vi "FPGAcode4_multipleArrays.vi"() -> ()   [LabVIEW 2015]
uses:
  Limits_In.ctl
  Detector_Cluster.ctl
  <vilib>/Platform/TimedLoop/XDataNode/timing_clust.ctl
  <vilib>/Platform/TimedLoop/XDataNode/nitl_modes.ctl
  <vilib>/Platform/TimedLoop/XDataNode/wakeup.ctl
  Correlations.ctl
  <vilib>/rvi/Emulation/niFpgaSctlEmulationGetInTimedLoop.vi
  <vilib>/rvi/Emulation/niFpgaEmulationReportErrorSimple.vi
  <vilib>/rvi/Emulation/niFpgaGetClockAttributes.vi
  <vilib>/rvi/Emulation/niFpgaCriticalErrorInLSC.vi
  <vilib>/rvi/eio/common/nirviEmuTemplateMethod_errors.vi
  <vilib>/rvi/Emulation/niFpgaEmulationIsFPGAContextNoSignature.vi
  <vilib>/rvi/DataTransferAndStorage/Container/Common/niFpgaContainerGetUniqueNameForEmu.vi
  <vilib>/rvi/eio/common/nirviEmuReportErrorAndStop.vi
  <vilib>/rvi/Emulation/niFpgaProcessEmulError.vi
  <vilib>/Platform/TimedLoop/XDataNode/XDataNode.xnode
  <vilib>/eio/EIONode/EIONode.xnode
  <vilib>/rvi/DataTransferAndStorage/Container/XNode/niFpgaContainer.xnode
  <vilib>/rvi/DataTransferAndStorage/Handshake/Emulation/niFpgaHandshakeEmulation.vi
  <vilib>/Platform/TimedLoop/XDataNode/XDNodeRunTimeDep.lvlib
panel:
  in  "Charge Error Factor":fxp<+,32,0>=0.19999999995343387 format="%_2g"
  in  "Calibrate":bool=TRUE
  in  "Limits":T1={"High Charge Limit"=4.54747350780585e-13, "Low Charge Limit"=0.0, "High Velocity Limit"=262143.0, "Low Velocity Limit"=0.0, "High Mass Limit"=7.27595761248936e-12, "Low Mass Limit"=0.0, "High Voltage"=2200000.0}
  in  "One Shot":bool
  in  "Threshold Factor":fxp<+/-,32,16>=1.149993896484375 format="%.2g"
  in  "Armed":bool
  in  "User Trigger Distance":fxp<+/-,34,18> format="%.3g"
  in  "User Trigger?":bool
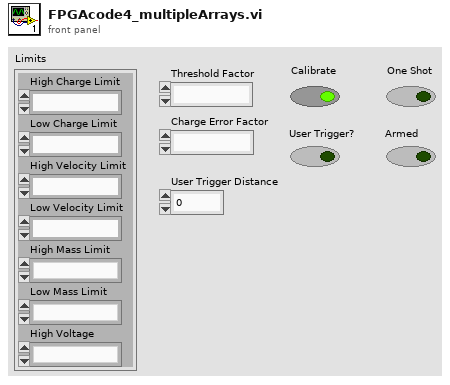
[diagram p1: front panel]
types:
  T1 = typedef "Limits_In.ctl" = cluster{"High Charge Limit":fxp<+,32,-41>, "Low Charge Limit":fxp<+,32,-41>, "High Velocity Limit":fxp<+,18,18>, "Low Velocity Limit":fxp<+,18,18>, "High Mass Limit":fxp<+,32,-37>, "Low Mass Limit":fxp<+,32,-37>, "High Voltage":fxp<+,32,22>}
  T2 = cluster{"[0]":fxp<+,16,1>, "[1]":fxp<+,16,1>, "[2]":fxp<+,16,1>, "[3]":fxp<+,16,1>, "[4]":fxp<+,16,1>, "[5]":fxp<+,16,1>, "[6]":fxp<+,16,1>, "[7]":fxp<+,16,1>, "[8]":fxp<+,16,1>, "[9]":fxp<+,16,1>, "[10]":fxp<+,16,1>}
  T3 = cluster{"[0]":i32, "[1]":i32, "[2]":i32, "[3]":i32, "[4]":i32, "[5]":i32, "[6]":i32, "[7]":i32, "[8]":i32, "[9]":i32, "[10]":i32}
  T4 = cluster{"[0]":cluster{"Detector Max Speed Count":i32, "Detector Min Speed Count":i32, "Gap Max Speed Count":i32, "Gap Min Speed Count":i32}, "[1]":cluster{"Detector Max Speed Count":i32, "Detector Min Speed Count":i32, "Gap Max Speed Count":i32, "Gap Min Speed Count":i32}, "[2]":cluster{"Detector Max Speed Count":i32, "Detector Min Speed Count":i32, "Gap Max Speed Count":i32, "Gap Min Speed Count":i32}, "[3]":cluster{"Detector Max Speed Count":i32, "Detector Min Speed Count":i32, "Gap Max Speed Count":i32, "Gap Min Speed Count":i32}, "[4]":cluster{"Detector Max Speed Count":i32, "Detector Min Speed Count":i32, "Gap Max Speed Count":i32, "Gap Min Speed Count":i32}, "[5]":cluster{"Detector Max Speed Count":i32, "Detector Min Speed Count":i32, "Gap Max Speed Count":i32, "Gap Min Speed Count":i32}, "[6]":cluster{"Detector Max Speed Count":i32, "Detector Min Speed Count":i32, "Gap Max Speed Count":i32, "Gap Min Speed Count":i32}, "[7]":cluster{"Detector Max Speed Count":i32, "Detector Min Speed Count":i32, "Gap Max Speed Count":i32, "Gap Min Speed Count":i32}, "[8]":cluster{"Detector Max Speed Count":i32, "Detector Min Speed Count":i32, "Gap Max Speed Count":i32, "Gap Min Speed Count":i32}, "[9]":cluster{"Detector Max Speed Count":i32, "Detector Min Speed Count":i32, "Gap Max Speed Count":i32, "Gap Min Speed Count":i32}, "[10]":cluster{"Detector Max Speed Count":i32, "Detector Min Speed Count":i32, "Gap Max Speed Count":i32, "Gap Min Speed Count":i32}}
  T5 = cluster{cluster{"[0]":i32, "[1]":i32, "[2]":i32, "[3]":i32, "[4]":i32, "[5]":i32, "[6]":i32, "[7]":i32, "[8]":i32, "[9]":i32, "[10]":i32}, cluster{"[0]":i32, "[1]":i32, "[2]":i32, "[3]":i32, "[4]":i32, "[5]":i32, "[6]":i32, "[7]":i32, "[8]":i32, "[9]":i32, "[10]":i32}, cluster{"[0]":i32, "[1]":i32, "[2]":i32, "[3]":i32, "[4]":i32, "[5]":i32, "[6]":i32, "[7]":i32, "[8]":i32, "[9]":i32, "[10]":i32}, cluster{"[0]":i32, "[1]":i32, "[2]":i32, "[3]":i32, "[4]":i32, "[5]":i32, "[6]":i32, "[7]":i32, "[8]":i32, "[9]":i32, "[10]":i32}}
  T6 = cluster{"Distance to PSU":fxp<+/-,64,37>, "Distance to end of PSU":fxp<+/-,64,37>, "Distance to DCS 2":fxp<+/-,64,37>, "Distance to DCS 1":fxp<+/-,64,37>, "Distance to front of LEIL Chamber":fxp<+/-,64,37>}
  T7 = typedef "Detector_Cluster.ctl" = cluster{"Det 1":i32, "Det 2":i32}
  T8 = cluster{"Filter 1":T7, "Filter 2":T7, "Filter 3":T7, "Filter 4":T7}
  T9 = cluster{"Detector Max Speed Count":i32, "Detector Min Speed Count":i32, "Gap Max Speed Count":i32, "Gap Min Speed Count":i32}[]
  T10 = cluster{"Filter 1":T7, "Filter 2":T7, "Filter 3":T7, "Filter 4":T7}[]
  T11 = typedef "XDNodeRunTimeDep.lvlib/timing_clust.ctl" = cluster{"Expected End [f-1]":u64, "Actual End [f-1]":u64, "Finished Late? [f-1]":bool, "Expected End [i-1]":u64, "Actual End [i-1]":u64, "Finished Late? [i-1]":bool, "Expected Start [i]":u64, "Actual Start [i]":u64, "Expected Start [f]":u64, "Actual Start [f]":u64, "Source Name":string, "Structure Name":string, "Period":i64, "Deadline":i64, "Offset":i64, "Start":i64, "Priority":i32, "Timeout":i32, "Mode":T12, "Wakeup Reason":T13, "Error":errorcluster, "Source Type":string, "Secondary Source Type":string, "Global End Time":u64, "Global Start Time":u64, "Frame Duration":u64, "Iteration Duration":u64, "Assigned CPU":i32, "I/O Scan Engine Mode":u32}
  T12 = typedef "XDNodeRunTimeDep.lvlib/nitl_modes.ctl" = enum32{"No Change", "Process missed periods, maintain original phase", "Discard missed periods, maintain original phase", "Process missed periods, ignore original phase", "Discard missed periods, ignore original phase"}
  T13 = typedef "XDNodeRunTimeDep.lvlib/wakeup.ctl" = enum32{"Normal", "Aborted", "Asynchronous wakeup", "Timing source error", "Timed loop error", "Timeout"}
  T14 = cluster{"IO Module\\AI 0":i16, "IO Module\\AI 1":i16}
  T15 = cluster{"First Detector Count":i32, "Detector Gap Count":i32, "Second Detector Count":i32, "Second Detector Final Count":i32}
  T16 = typedef "Correlations.ctl" = cluster{"First Correlation":i32, "Latest Correlation":i32}
  T17 = cluster{"Data":fxp<+/-,40,32>, "Data":fxp<+/-,40,32>}
  T18 = cluster{cluster{"Data":i16, "Data":i16}, cluster{"Det 1":i16, "Det 2":i16}, cluster{"Det 1":i16, "Det 2":i16}, cluster{"Det 1":i16, "Det 2":i16}}
  T19 = cluster{cluster{"Det 1":i16, "Det 2":i16}, cluster{"Det 1":i16, "Det 2":i16}, cluster{"Det 1":i16, "Det 2":i16}, cluster{"Det 1":i16, "Det 2":i16}}
  T20 = cluster{"Distance to PSU":fxp<+/-,64,69>, "Distance to end of PSU":fxp<+/-,64,69>, "Distance to DCS 2":fxp<+/-,64,69>, "Distance to DCS 1":fxp<+/-,64,69>, "Distance to front of LEIL Chamber":fxp<+/-,64,69>}
  T21 = cluster{"Distance to PSU":i32, "Distance to end of PSU":i32, "Distance to DCS 2":i32, "Distance to DCS 1":i32, "Distance to front of LEIL Chamber":i32}
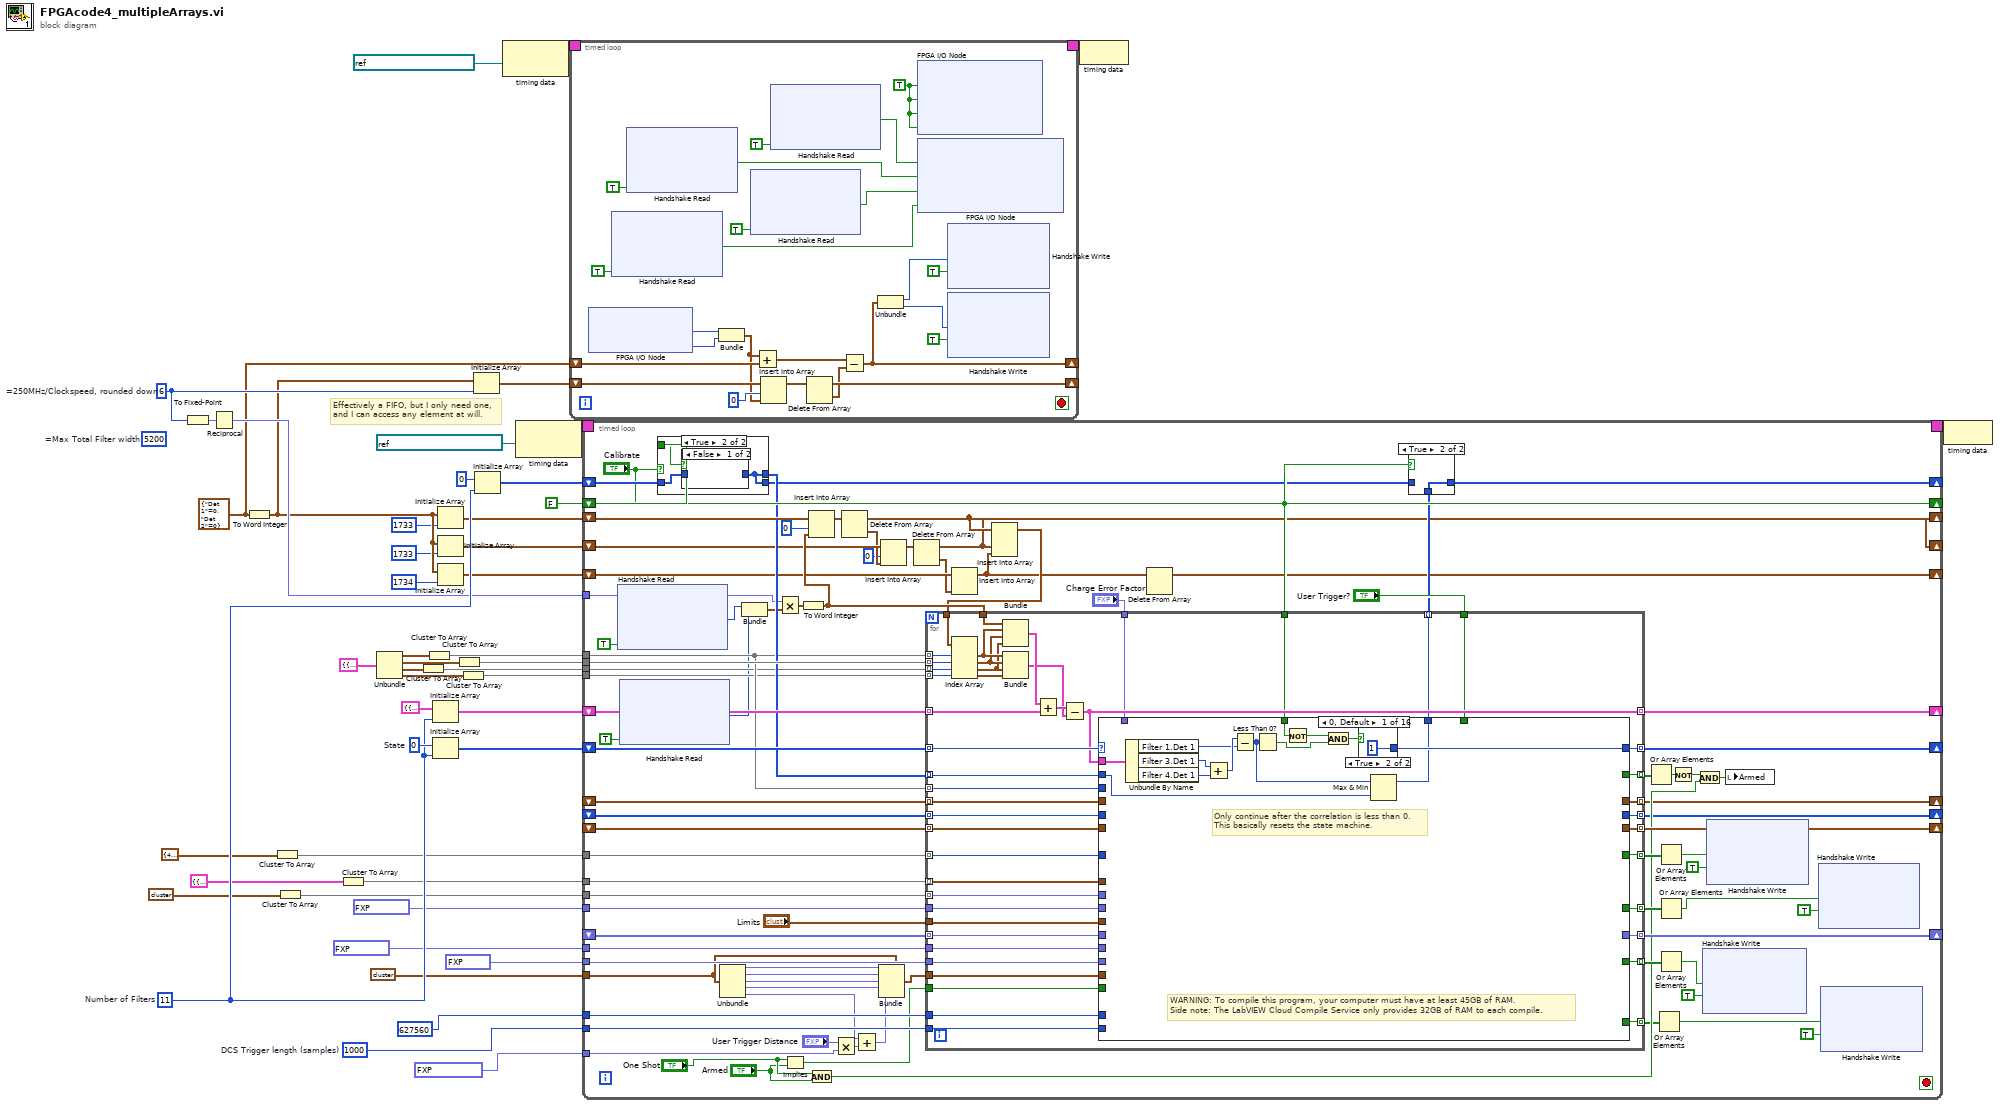
[diagram p0: block diagram]
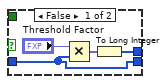
[diagram p2: hidden frame]
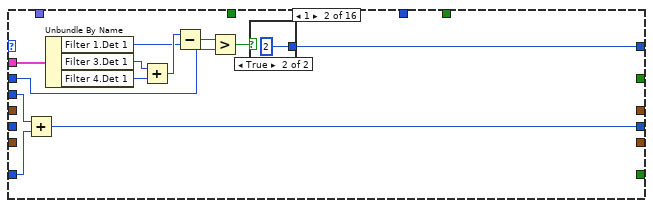
[diagram p6: hidden frame]
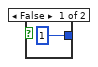
[diagram p7: hidden frame]
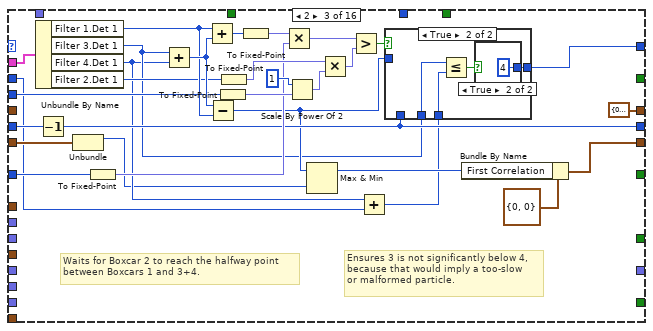
[diagram p8: hidden frame]
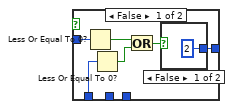
[diagram p9: hidden frame]
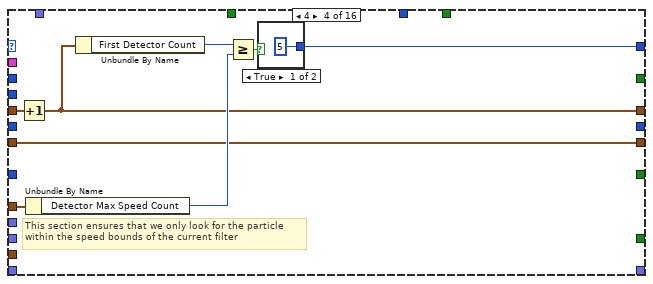
[diagram p12: hidden frame]
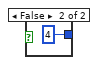
[diagram p13: hidden frame]
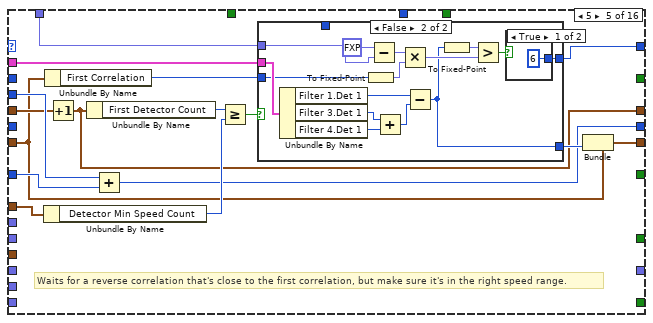
[diagram p14: hidden frame]
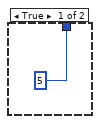
[diagram p15: hidden frame]
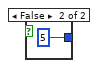
[diagram p16: hidden frame]
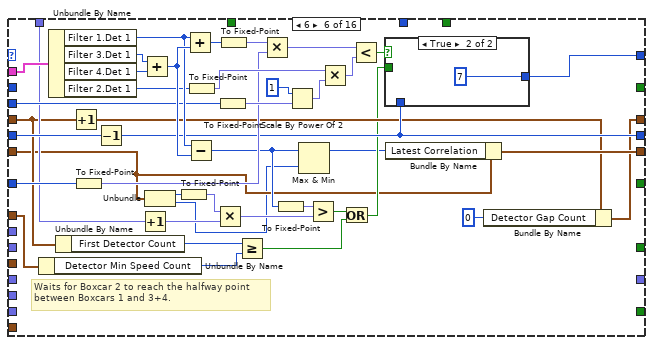
[diagram p17: hidden frame]
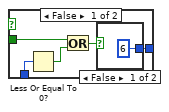
[diagram p18: hidden frame]
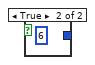
[diagram p19: hidden frame]
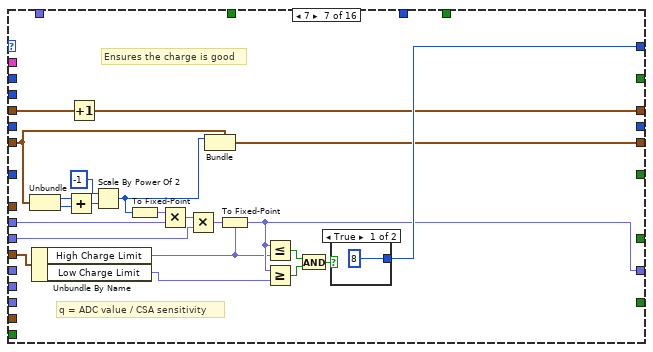
[diagram p20: hidden frame]
diagram:
  w40 = u8 6  # =250MHz/Clockspeed, rounded down
  (unwired) 5200  # =Max Total Filter width
  w10 = u16 1000  # DCS Trigger length (samples)
  w7 = T7 {"Det 1"=0, "Det 2"=0} ("Detectors")
  w48 = u8 0  # State
  w45 = 11  # Number of Filters
  # "Effectively a FIFO, but I only need one,\nand I can access any element at will."
  n1 = To Fixed-Point(number=w40) -> (fixed-point=w42:fxp<+,8,8>)  [unwired: 1 in]
  n2 = Reciprocal(x=w42) -> (1/x=w25:fxp<+,9,1>)
  n3 = To Word Integer(number=w7) -> (16bit integer=w6:cluster{"Det 1":i16, "Det 2":i16})
  n4 = Cluster To Array(cluster=T3 {"[0]"=4000, "[1]"=2359, "[2]"=1391, "[3]"=820, "[4]"=484, "[5]"=285, "[6]"=168, "[7]"=99, "[8]"=59, "[9]"=35, "[10]"=20}) -> (array=w18:i32[])
  n5 = Cluster To Array(cluster=T2 {"[0]"=0.000823974609375, "[1]"=0.000823974609375, "[2]"=0.000823974609375, "[3]"=0.000823974609375, "[4]"=0.000823974609375, "[5]"=0.00152587890625, "[6]"=0.003265380859375, "[7]"=0.007080078125, "[8]"=0.015869140625, "[9]"=0.03704833984375, "[10]"=0.100006103515625} ("cluster 3")) -> (array=w16:fxp<+,16,1>[])
  n6 = Cluster To Array(cluster=T4 {"[0]"={"Detector Max Speed Count"=42000, "Detector Min Speed Count"=84000, "Gap Max Speed Count"=78000, "Gap Min Speed Count"=156000}, "[1]"={"Detector Max Speed Count"=21477, "Detector Min Speed Count"=42953, "Gap Max Speed Count"=39885, "Gap Min Speed Count"=79770}, "[2]"={"Detector Max Speed Count"=10982, "Detector Min Speed Count"=21964, "Gap Max Speed Count"=20395, "Gap Min Speed Count"=40790}, "[3]"={"Detector Max Speed Count"=5616, "Detector Min Speed Count"=11231, "Gap Max Speed Count"=10429, "Gap Min Speed Count"=20858}, "[4]"={"Detector Max Speed Count"=2872, "Detector Min Speed Count"=5743, "Gap Max Speed Count"=5333, "Gap Min Speed Count"=10666}, "[5]"={"Detector Max Speed Count"=1468, "Detector Min Speed Count"=2937, "Gap Max Speed Count"=2727, "Gap Min Speed Count"=5454}, "[6]"={"Detector Max Speed Count"=751, "Detector Min Speed Count"=1502, "Gap Max Speed Count"=1394, "Gap Min Speed Count"=2789}, "[7]"={"Detector Max Speed Count"=384, "Detector Min Speed Count"=768, "Gap Max Speed Count"=713, "Gap Min Speed Count"=1426}, "[8]"={"Detector Max Speed Count"=196, "Detector Min Speed Count"=393, "Gap Max Speed Count"=365, "Gap Min Speed Count"=729}, "[9]"={"Detector Max Speed Count"=100, "Detector Min Speed Count"=201, "Gap Max Speed Count"=186, "Gap Min Speed Count"=373}, "[10]"={"Detector Max Speed Count"=51, "Detector Min Speed Count"=103, "Gap Max Speed Count"=95, "Gap Min Speed Count"=191}} ("cluster 2")) -> (array=w17:T9)
  n7 = Unbundle(T5 {{"[0]"=1200, "[1]"=1200, "[2]"=1200, "[3]"=1200, "[4]"=1200, "[5]"=650, "[6]"=306, "[7]"=140, "[8]"=62, "[9]"=26, "[10]"=10}, {"[0]"=5200, "[1]"=3559, "[2]"=2591, "[3]"=2020, "[4]"=1684, "[5]"=935, "[6]"=474, "[7]"=240, "[8]"=122, "[9]"=62, "[10]"=30}, {"[0]"=5800, "[1]"=4159, "[2]"=3191, "[3]"=2620, "[4]"=2284, "[5]"=1260, "[6]"=627, "[7]"=310, "[8]"=153, "[9]"=75, "[10]"=35}, {"[0]"=6400, "[1]"=4759, "[2]"=3791, "[3]"=3220, "[4]"=2884, "[5]"=1585, "[6]"=780, "[7]"=380, "[8]"=184, "[9]"=88, "[10]"=40}} ("output cluster")) -> (w38:T3, w37:T3, w36:T3, w35:T3)
  n8 = Cluster To Array(cluster=w36) -> (array=w22:i32[])
  n9 = Cluster To Array(cluster=w38) -> (array=w24:i32[])
  n10 = Initialize Array(T8 {"Filter 1"={"Det 1"=0, "Det 2"=0}, "Filter 2"={"Det 1"=0, "Det 2"=0}, "Filter 3"={"Det 1"=0, "Det 2"=0}, "Filter 4"={"Det 1"=0, "Det 2"=0}} ("cluster"), w45) -> (w20:T10)
  n11 = Initialize Array(w48, w45) -> (w19:u8[])
  n12 = Initialize Array(w6, 1733 ("dimension size")) -> (w26:cluster{"Det 1":i16, "Det 2":i16}[])
  n13 = Initialize Array(w6, 1733 ("dimension size")) -> (w5:cluster{"Det 1":i16, "Det 2":i16}[])
  n14 = Initialize Array(w6, 1734 ("dimension size")) -> (w4:cluster{"Det 1":i16, "Det 2":i16}[])
  n15 = Cluster To Array(cluster=w37) -> (array=w23:i32[])
  n16 = Cluster To Array(cluster=w35) -> (array=w21:i32[])
  n17 = Initialize Array(w6, w40) -> (w41:cluster{"Det 1":i16, "Det 2":i16}[])
  n18 = Initialize Array(0 ("Thresholds in"), w45) -> (w27:i32[])
  n19 = node-c288(refnum<k21> "IO Module\\Data Clock" ("Source Name")) -> (w44:T11)
  n20 = node-c288(refnum<k21> "40 MHz Onboard Clock" ("Source Name")) -> (w30:T11)
  n21 = timed-loop {
    timing: w44 -> [_]
    timing-out: [_] -> w43
    shift-right: [w62] -> _
    shift-left: w7 -> [w71]
    shift-right: [w64] -> _
    shift-left: w41 -> [w69]
    stop <- _ stop-if-true
    w49 = TRUE ("IO Module\\PFI Enable")
    n22 = xnode "FPGA I/O Node"() -> ("IO Module\\AI 0"=w68:i16, "IO Module\\AI 1"=w67:i16)  [unwired: 2 in, 2 out]
    n23 = xnode ("Handshake Read")("Ready for Output"=TRUE) -> ("Data"=w57:bool)  [unwired: 1 in, 2 out]
    n24 = xnode ("Handshake Read")("Ready for Output"=TRUE) -> ("Data"=w53:bool)  [unwired: 1 in, 2 out]
    n25 = Bundle("IO Module\\AI 0"=w68, "IO Module\\AI 1"=w67) -> (w66:T14)  [unwired: 1 in]
    n26 = xnode ("Handshake Read")("Ready for Output"=TRUE) -> ("Data"=w56:bool)  [unwired: 1 in, 2 out]
    n27 = Add(x=w66, y=w71) -> (x+y=w70:T7)
    n28 = Insert Into Array(array=w69, index=0, new element=w66) -> (w65:cluster{"Det 1":i16, "Det 2":i16}[])
    n29 = xnode ("Handshake Read")("Ready for Output"=TRUE) -> ("Data"=w50:bool)  [unwired: 1 in, 2 out]
    n30 = Delete From Array(array=w65) -> (deleted portion=w63:cluster{"Det 1":i16, "Det 2":i16}, array with subset deleted=w64:cluster{"Det 1":i16, "Det 2":i16}[])  [unwired: 2 in]
    n31 = Subtract(x=w70, y=w63) -> (x-y=w62:T7)
    n32 = Unbundle(w62) -> ("Det 1"=w60:i32, "Det 2"=w58:i32)
    n33 = xnode "FPGA I/O Node"("IO Module\\PFI 0 WE"=w49, "IO Module\\PFI 1 WE"=w49, "IO Module\\PFI 2 WE"=w49, "IO Module\\PFI 3 WE"=w49) -> ()  [unwired: 4 in, 4 out]
    n34 = xnode "FPGA I/O Node"("IO Module\\PFI 0 Wr Data"=w50, "IO Module\\PFI 1 Wr Data"=w53, "IO Module\\PFI 2 Wr Data"=w56, "IO Module\\PFI 3 Wr Data"=w57) -> ()  [unwired: 4 in, 4 out]
    n35 = xnode ("Handshake Write")("Data"=w60, "Input Valid"=TRUE) -> ()  [unwired: 1 in, 2 out]
    n36 = xnode ("Handshake Write")("Data"=w58, "Input Valid"=TRUE) -> ()  [unwired: 1 in, 2 out]
  }
  n37 = timed-loop {
    shift-right: [w80] -> _
    shift-left: w26 -> [w161]
    shift-right: [w111] -> _
    shift-left: w20 -> [w158]
    shift-right: [w105] -> _
    shift-left: w19 -> [w160]
    shift-right: [w112] -> _
    shift-left: _ -> [w159]
    tunnel: w17 -> [w157]
    shift-right: [w156] -> _
    shift-left: _ -> [w155]
    tunnel: w24 -> [w110]
    tunnel: w23 -> [w154]
    tunnel: w18 -> [w153]
    tunnel: w16 -> [w152]
    shift-right: [w151] -> _
    shift-left: _ -> [w150]
    tunnel: fxp<+,32,-43> 9.525990075777386e-16 ("fixed-point 2") -> [w149]
    tunnel: fxp<+,32,-49> 2.2727300016438096e-16 ("fixed-point 3") -> [w148]
    tunnel: fxp<+,28,28> 32400000.0 ("fixed-point") -> [w147]
    tunnel: T6 {"Distance to PSU"=1.2345678955316544, "Distance to end of PSU"=2.4691357985138893, "Distance to DCS 2"=3.229876533150673, "Distance to DCS 1"=-1.677654318511486, "Distance to front of LEIL Chamber"=5.305777758359909} ("x/y") -> [w140]
    shift-right: [w146] -> _
    shift-left: w27 -> [w145]
    shift-right: ["Calibrate"] -> _
    shift-left: FALSE ("Calibrate") -> [w144]
    tunnel: w10 -> [w143]
    tunnel: 627560 ("32bit integer") -> [w142]
    tunnel: fxp<+,32,1> 1.2345679011195898 ("1/x") -> [w141]
    shift-right: [w109] -> _
    shift-left: _ -> [w108]
    tunnel: w21 -> [w107]
    tunnel: w22 -> [w106]
    timing: w30 -> [_]
    timing-out: [_] -> w29
    tunnel: w25 -> [w103]
    shift-right: [w75] -> _
    shift-left: w5 -> [w86]
    shift-right: [w76] -> _
    shift-left: w4 -> [w85]
    stop <- _ stop-if-true
    n38 = xnode ("Handshake Read")("Ready for Output"=TRUE) -> ("Data"=w90:i32)  [unwired: 1 in, 2 out]
    n39 = xnode ("Handshake Read")("Ready for Output"=TRUE) -> ("Data"=w89:i32)  [unwired: 1 in, 2 out]
    n40 = case shown="True" "Calibrate" {
      tunnel: w145 -> [w163 w167]
      tunnel: [w163 w166] -> w113
      tunnel: w144 -> [_ w168]
      tunnel: [w162 w166] -> w114
      frame False {
        n41 = Multiply(x="Threshold Factor", y=w163) -> (x*y=w164:fxp<+/-,64,48>[])
        n42 = To Long Integer(number=w164) -> (32bit integer=w162:i32[])
      }
      frame True {
        n43 = case shown="False" w168 {
          tunnel: w167 -> [_ w169]
          tunnel: [_ w169] -> w166
          frame False {
          }
          frame True {
          }
        }
      }
    }
    n44 = Unbundle(w140) -> ("Distance to PSU"=w134:fxp<+/-,64,37>, "Distance to end of PSU"=w133:fxp<+/-,64,37>, "Distance to DCS 2"=w132:fxp<+/-,64,37>, "Distance to DCS 1"=w129:fxp<+/-,64,37>, "Distance to front of LEIL Chamber"=w128:fxp<+/-,64,37>)
    n45 = Bundle("Data"=w90, "Data"=w89) -> (w88:cluster{"Data":i32, "Data":i32})  [unwired: 1 in]
    n46 = Multiply(x=w103, y=w88) -> (x*y=w104:T17)
    n47 = Implies(1:"Armed", 2:"One Shot") -> (0:w136:bool)
    n48 = To Word Integer(number=w104) -> (16bit integer=w102:cluster{"Data":i16, "Data":i16})
    n49 = Insert Into Array(array=w161, index=0, new element=w102) -> (w79:cluster{"Det 1":i16, "Det 2":i16}[])
    n50 = And(x="One Shot", y="Armed") -> (x .and. y?=w120:bool)
    n51 = Multiply(x="User Trigger Distance", y=w141) -> (x*y=w130:fxp<+/-,64,18>)
    n52 = Delete From Array(array=w79) -> (deleted portion=w84:cluster{"Det 1":i16, "Det 2":i16}, array with subset deleted=w80:cluster{"Det 1":i16, "Det 2":i16}[])  [unwired: 2 in]
    n53 = Add(x=w128, y=w130) -> (x+y=w127:fxp<+/-,64,38>)
    n54 = Bundle(cluster=w140, "Distance to PSU"=w134, "Distance to end of PSU"=w133, "Distance to DCS 2"=w132, "Distance to DCS 1"=w129, "Distance to front of LEIL Chamber"=w127) -> (w131:T6)
    n55 = Insert Into Array(array=w86, index=0, new element=w84) -> (w83:cluster{"Det 1":i16, "Det 2":i16}[])
    n56 = Delete From Array(array=w83) -> (deleted portion=w82:cluster{"Det 1":i16, "Det 2":i16}, array with subset deleted=w75:cluster{"Det 1":i16, "Det 2":i16}[])  [unwired: 2 in]
    n57 = Insert Into Array(array=w85, new element=w82) -> (w77:cluster{"Det 1":i16, "Det 2":i16}[])  [unwired: 1 in]
    n58 = Insert Into Array(array=w80, new element #1=w75, new element #2=w77) -> (w78:cluster{"Det 1":i16, "Det 2":i16}[])  [unwired: 1 in]
    n59 = for {
      tunnel: w78 -> [w218]
      tunnel: [w204] -> w111 mode=indexing
      tunnel: w160 -> [w217] mode=indexing
      tunnel: [w216] -> w105 mode=indexing
      tunnel: w114 -> [w177] mode=indexing
      tunnel: [w215] -> w112 mode=indexing
      tunnel: w159 -> [w214] mode=indexing
      tunnel: w158 -> [w208] mode=indexing
      tunnel: w102 -> [w213]
      tunnel: w157 -> [w203] mode=indexing
      tunnel: [w202] -> w156 mode=indexing
      tunnel: w155 -> [w201] mode=indexing
      tunnel: w110 -> [w200] mode=indexing
      tunnel: w154 -> [w175] mode=indexing
      tunnel: w106 -> [w199] mode=indexing
      tunnel: w107 -> [w198] mode=indexing
      tunnel: w110 -> [w179] mode=indexing
      tunnel: w153 -> [w178] mode=indexing
      tunnel: "Charge Error Factor" -> [w197]
      tunnel: w152 -> [w196] mode=indexing
      tunnel: "Limits" -> [w195]
      tunnel: [w194] -> w151 mode=indexing
      tunnel: w150 -> [w193] mode=indexing
      tunnel: w149 -> [w192]
      tunnel: w148 -> [w191]
      tunnel: w147 -> [w190]
      tunnel: w131 -> [w189]
      tunnel: w136 -> [w188]
      tunnel: w143 -> [w186]
      tunnel: w142 -> [w187]
      tunnel: [w185] -> w126 mode=indexing
      tunnel: [w184] -> w125 mode=indexing
      tunnel: [w183] -> w124 mode=indexing
      tunnel: [w182] -> w123 mode=indexing
      tunnel: "User Trigger?" -> [w181]
      tunnel: "Calibrate" -> [w180]
      tunnel: [w176] -> w109 mode=indexing
      tunnel: w108 -> [w174] mode=indexing
      tunnel: [w173] -> w101 mode=indexing
      tunnel: [w172] -> w87 mode=indexing
      n60 = Index Array(array=w218, index #1=w200, index #2=w175, index #3=w199, index #4=w198) -> (element #1=w211:cluster{"Det 1":i16, "Det 2":i16}, element #2=w210:cluster{"Det 1":i16, "Det 2":i16}, element #3=w209:cluster{"Det 1":i16, "Det 2":i16}, element #4=w212:cluster{"Det 1":i16, "Det 2":i16})
      n61 = Bundle(w213, w211, w210, w209) -> (w207:T18)  [unwired: 1 in]
      n62 = Bundle(w211, w210, w209, w212) -> (w205:T19)  [unwired: 1 in]
      n63 = Add(x=w207, y=w208) -> (x+y=w206:T8)
      n64 = Subtract(x=w206, y=w205) -> (x-y=w204:T8)
      n65 = case shown="0, Default" w217 {
        tunnel: w177 -> [w221 w244 w250 _ _ _ _ _ _ _ _ _ _ _ _ _]
        tunnel: [w230 w243 w275 w292 w307 w373 w395 w409 w423 w486 w499 w513 w574 w601 u8 16 ("Det 3") w665] -> w216
        tunnel: w179 -> [_ w236 w269 _ w309 w365 _ _ w425 w478 _ w515 w566 _ w633 _]
        tunnel: [_ _ T15 {"First Detector Count"=0, "Detector Gap Count"=0, "Second Detector Count"=0, "Second Detector Final Count"=0} ("Cutoffs") w289 w299 w336 w385 w406 w417 w450 w496 w508 w554 w584 w624 w663] -> w215
        tunnel: w214 -> [_ _ _ w290 w304 w341 w386 w407 w420 w456 w497 w510 w544 w584 w623 w664]
        tunnel: w174 -> [_ _ w276 _ _ w374 _ _ _ w487 _ _ w575 _ _ w646]
        tunnel: w204 -> [w225 w238 w262 _ w310 w358 _ _ w426 w472 _ w516 w560 _ _ _]
        tunnel: w203 -> [_ _ _ w296 w314 w342 _ w413 w430 w455 w503 w520 w545 _ _ _]
        tunnel: w201 -> [_ _ w253 w291 w301 w340 w388 w408 w419 w465 w498 w506 w538 _ _ _]
        tunnel: w178 -> [_ w235 w270 _ w308 w366 _ _ w424 w479 _ w514 w567 _ w627 _]
        tunnel: w197 -> [_ _ _ _ w311 w351 _ _ w427 w466 _ w517 w553 _ _ _]
        tunnel: w196 -> [_ _ _ _ _ _ w400 _ _ _ _ _ _ _ _ _]
        tunnel: w195 -> [_ _ _ _ _ _ w403 _ _ _ _ _ _ w612 _ _]
        tunnel: [_ _ _ _ _ _ w383 w405 w416 w448 w495 w507 w539 _ _ _] -> w194
        tunnel: w193 -> [_ _ _ _ _ _ _ w405 w416 w448 w495 w507 w539 w590 _ _]
        tunnel: w192 -> [_ _ _ _ _ _ _ _ _ _ _ _ _ w611 _ _]
        tunnel: w191 -> [_ _ _ _ _ _ w393 _ _ _ _ _ _ _ _ _]
        tunnel: w190 -> [_ _ _ _ _ _ _ _ _ _ _ _ _ w589 _ _]
        tunnel: w189 -> [_ _ _ _ _ _ _ _ _ _ _ _ _ _ w636 _]
        tunnel: w188 -> [_ _ _ _ _ _ _ _ _ _ _ _ _ w595 _ _]
        tunnel: w187 -> [_ _ _ _ _ _ _ _ _ _ _ _ _ _ w630 _]
        tunnel: w186 -> [_ _ _ _ _ _ _ _ _ _ _ _ _ _ _ w643]
        tunnel: [_ _ _ _ _ _ _ _ _ _ _ _ _ _ _ w662] -> w185
        tunnel: [_ _ _ _ _ _ _ _ _ _ _ _ _ _ _ w661] -> w184
        tunnel: [_ _ _ _ _ _ _ _ _ _ _ _ _ _ _ w645] -> w183
        tunnel: [_ _ _ _ _ _ _ _ _ _ _ _ _ w594 _ _] -> w182
        tunnel: w181 -> [_ _ _ _ _ _ _ _ _ _ _ _ _ _ _ w647]
        tunnel: w180 -> [w223 _ _ _ _ _ _ _ _ _ _ _ _ _ _ _]
        tunnel: [_ w234 w258 _ w300 w354 _ _ w418 w468 _ w509 w556 _ _ w639] -> w176
        tunnel: [_ _ w264 w291 w303 w360 w387 w408 w419 w465 w498 w506 w538 _ _ _] -> w202
        tunnel: [w219 _ _ _ _ _ _ _ _ _ _ _ _ _ _ _] -> w173
        tunnel: [_ _ _ _ _ _ _ _ _ _ _ _ _ _ _ w644] -> w172
        frame 0, Default {
          # "WARNING: To compile this program, your computer must have at least 45GB of RAM.\nSide note: The LabVIEW Cloud Compile Service only provides 32GB of RAM to each compile."
          # "Only continue after the correlation is less than 0.\nThis basically resets the state machine."
          n66 = Unbundle By Name(w225) -> ("Filter 1.Det 1"=w226:i32, "Filter 3.Det 1"=w227:i32, "Filter 4.Det 1"=w228:i32)
          n67 = Add(x=w227, y=w228) -> (x+y=w229:i32)
          n68 = Subtract(x=w229, y=w226) -> (x-y=w220:i32)
          n69 = Less Than 0?(x=w220) -> (x < 0?=w231:bool)
          n70 = Not(x=w223) -> (.not. x?=w222:bool)
          n71 = And(x=w222, y=w231) -> (x .and. y?=w224:bool)
          n72 = case shown="True" w224 {
            tunnel: [_ u8 1 ("Det 3")] -> w230
            frame False {
            }
            frame True {
            }
          }
          n73 = Max & Min(x=w220, y=w221) -> (max(x,y)=w219:i32)  [unwired: 1 out]
        }
        frame 1 {
          n74 = Add(x=w236, y=w235) -> (x+y=w234:i32)
          n75 = Unbundle By Name(w238) -> ("Filter 1.Det 1"=w239:i32, "Filter 3.Det 1"=w240:i32, "Filter 4.Det 1"=w241:i32)
          n76 = Add(x=w240, y=w241) -> (x+y=w242:i32)
          n77 = Subtract(x=w242, y=w239) -> (x-y=w237:i32)
          n78 = Greater?(x=w237, y=w244) -> (0:w233:bool)
          n79 = case shown="True" w233 {
            tunnel: [u8 1 ("Det 3") u8 2 ("Det 3")] -> w243
            frame False {
            }
            frame True {
            }
          }
        }
        frame 2 {
          # "Ensures 3 is not significantly below 4,\nbecause that would imply a too-slow\nor malformed particle."
          # "Waits for Boxcar 2 to reach the halfway point\nbetween Boxcars 1 and 3+4."
          n80 = Unbundle By Name(w262) -> ("Filter 1.Det 1"=w272:i32, "Filter 3.Det 1"=w249:i32, "Filter 4.Det 1"=w248:i32, "Filter 2.Det 1"=w266:i32)
          n81 = Decrement(x=w276) -> (x-1=w258:i32)
          n82 = Unbundle(w253) -> ("First Correlation"=w247:i32)  [unwired: 1 out]
          n83 = To Fixed-Point(number=w270) -> (fixed-point=w259:fxp<+/-,32,32>)  [unwired: 1 in]
          n84 = Add(x=w249, y=w248) -> (x+y=w273:i32)
          n85 = Add(x=w272, y=w273) -> (x+y=w274:i32)
          n86 = Subtract(x=w273, y=w272) -> (x-y=w254:i32)
          n87 = To Fixed-Point(number=w269) -> (fixed-point=w260:fxp<+/-,32,32>)  [unwired: 1 in]
          n88 = To Fixed-Point(number=w266) -> (fixed-point=w261:fxp<+/-,32,32>)  [unwired: 1 in]
          n89 = To Fixed-Point(number=w274) -> (fixed-point=w263:fxp<+/-,32,32>)  [unwired: 1 in]
          n90 = Multiply(x=w263, y=w259) -> (x*y=w271:fxp<+/-,64,64>)
          n91 = Scale By Power Of 2(n=i16 1, x=w260) -> (x*2^n=w267:fxp<+/-,32,32>)
          n92 = Max & Min(x=w254, y=w247) -> (max(x,y)=w255:i32)  [unwired: 1 out]
          n93 = Multiply(x=w261, y=w267) -> (x*y=w265:fxp<+/-,64,64>)
          n94 = Greater?(x=w271, y=w265) -> (0:w256:bool)
          n95 = Add(x=w248, y=w250) -> (x+y=w251:i32)
          n96 = case shown="True" w256 {
            tunnel: [w282 w287] -> w275
            tunnel: w258 -> [w278 _]
            tunnel: w254 -> [w277 _]
            tunnel: w251 -> [_ w285]
            tunnel: w249 -> [_ w286]
            frame False {
              n97 = Less Or Equal To 0?(x=w277) -> (x <= 0?=w280:bool)
              n98 = Less Or Equal To 0?(x=w278) -> (x <= 0?=w279:bool)
              n99 = Or(x=w280, y=w279) -> (x .or. y?=w281:bool)
              n100 = case shown="False" w281 {
                tunnel: [u8 2 ("Det 3") _] -> w282
                frame False {
                }
                frame True {
                }
              }
            }
            frame True {
              n101 = Less Or Equal?(x=w286, y=w285) -> (x <= y?=w284:bool)
              n102 = case shown="True" w284 {
                tunnel: [_ u8 4 ("Det 3")] -> w287
                frame False {
                }
                frame True {
                }
              }
            }
          }
          n103 = Bundle By Name(cluster=T16 {"First Correlation"=0, "Latest Correlation"=0}, "First Correlation"=w255) -> (w264:T16)
        }
        frame 4 {
          # "This section ensures that we only look for the particle\nwithin the speed bounds of the current filter"
          n104 = Increment(x=w290) -> (x+1=w289:T15)
          n105 = Unbundle By Name(w296) -> ("Detector Max Speed Count"=w294:i32)
          n106 = Unbundle By Name(w289) -> ("First Detector Count"=w295:i32)
          n107 = Greater Or Equal?(x=w295, y=w294) -> (x >= y?=w293:bool)
          n108 = case shown="True" w293 {
            tunnel: [u8 5 u8 4] -> w292
            frame True {
            }
            frame False {
            }
          }
        }
        frame 5 {
          # "Waits for a reverse correlation that's close to the first correlation, but make sure it's in the right speed range."
          n109 = Unbundle By Name(w314) -> ("Detector Min Speed Count"=w313:i32)
          n110 = Unbundle By Name(w301) -> ("First Correlation"=w306:i32)
          n111 = Increment(x=w304) -> (x+1=w299:T15)
          n112 = Unbundle By Name(w299) -> ("First Detector Count"=w305:i32)
          n113 = Add(x=w309, y=w308) -> (x+y=w300:i32)
          n114 = Greater Or Equal?(x=w305, y=w313) -> (x >= y?=w312:bool)
          n115 = case shown="False" w312 {
            tunnel: [_ w330] -> w307
            tunnel: [u8 5 _] -> _
            tunnel: w311 -> [_ w329]
            tunnel: w310 -> [_ w326]
            tunnel: w306 -> [_ w317]
            tunnel: [_ w316] -> w302
            frame True {
            }
            frame False {
              n116 = Unbundle By Name(w326) -> ("Filter 1.Det 1"=w323:i32, "Filter 3.Det 1"=w325:i32, "Filter 4.Det 1"=w324:i32)
              n117 = To Fixed-Point(number=w317) -> (fixed-point=w319:fxp<+/-,32,32>)  [unwired: 1 in]
              n118 = Subtract(x=fxp<+,1,1> 1.0, y=w329) -> (x-y=w327:fxp<+,33,1>)
              n119 = Add(x=w325, y=w324) -> (x+y=w322:i32)
              n120 = Multiply(x=w327, y=w319) -> (x*y=w321:fxp<+/-,64,32>)
              n121 = Subtract(x=w323, y=w322) -> (x-y=w316:i32)
              n122 = To Fixed-Point(number=w316) -> (fixed-point=w318:fxp<+/-,32,32>)  [unwired: 1 in]
              n123 = Greater?(x=w318, y=w321) -> (0:w320:bool)
              n124 = case shown="True" w320 {
                tunnel: [u8 6 u8 5] -> w330
                frame True {
                }
                frame False {
                }
              }
            }
          }
          n125 = Bundle(cluster=w301, "Latest Correlation"=w302) -> (w303:T16)  [unwired: 1 in]
        }
        frame 6 {
          # "Waits for Boxcar 2 to reach the halfway point\nbetween Boxcars 1 and 3+4."
          n126 = Unbundle By Name(w342) -> ("Detector Min Speed Count"=w338:i32)
          n127 = Unbundle By Name(w358) -> ("Filter 1.Det 1"=w368:i32, "Filter 3.Det 1"=w371:i32, "Filter 4.Det 1"=w370:i32, "Filter 2.Det 1"=w362:i32)
          n128 = Unbundle By Name(w341) -> ("First Detector Count"=w339:i32)
          n129 = Increment(x=w341) -> (x+1=w352:T15)
          n130 = To Fixed-Point(number=w366) -> (fixed-point=w355:fxp<+/-,32,32>)  [unwired: 1 in]
          n131 = Decrement(x=w374) -> (x-1=w354:i32)
          n132 = Increment(x=w351) -> (x+1=w348:fxp<+,33,1>)
          n133 = Add(x=w371, y=w370) -> (x+y=w369:i32)
          n134 = Unbundle(w340) -> ("First Correlation"=w350:i32, "Latest Correlation"=w334:i32)
          n135 = To Fixed-Point(number=w350) -> (fixed-point=w349:fxp<+/-,32,32>)  [unwired: 1 in]
          n136 = Add(x=w368, y=w369) -> (x+y=w372:i32)
          n137 = Subtract(x=w368, y=w369) -> (x-y=w347:i32)
          n138 = To Fixed-Point(number=w362) -> (fixed-point=w357:fxp<+/-,32,32>)  [unwired: 1 in]
          n139 = Multiply(x=w349, y=w348) -> (x*y=w345:fxp<+/-,64,33>)
          n140 = To Fixed-Point(number=w365) -> (fixed-point=w356:fxp<+/-,32,32>)  [unwired: 1 in]
          n141 = To Fixed-Point(number=w372) -> (fixed-point=w359:fxp<+/-,32,32>)  [unwired: 1 in]
          n142 = Greater Or Equal?(x=w339, y=w338) -> (x >= y?=w337:bool)
          n143 = Multiply(x=w359, y=w355) -> (x*y=w367:fxp<+/-,64,64>)
          n144 = To Fixed-Point(number=w347) -> (fixed-point=w346:fxp<+/-,32,32>)  [unwired: 1 in]
          n145 = Scale By Power Of 2(n=i16 1, x=w356) -> (x*2^n=w363:fxp<+/-,32,32>)
          n146 = Max & Min(x=w347, y=w334) -> (max(x,y)=w333:i32)  [unwired: 1 out]
          n147 = Greater?(x=w346, y=w345) -> (0:w344:bool)
          n148 = Multiply(x=w357, y=w363) -> (x*y=w361:fxp<+/-,64,64>)
          n149 = Or(x=w344, y=w337) -> (x .or. y?=w343:bool)
          n150 = Less?(x=w367, y=w361) -> (x < y?=w353:bool)
          n151 = case shown="True" w353 {
            tunnel: [w379 u8 7 ("Det 3")] -> w373
            tunnel: w354 -> [w376 _]
            tunnel: w343 -> [w375 _]
            frame False {
              n152 = Less Or Equal To 0?(x=w376) -> (x <= 0?=w377:bool)
              n153 = Or(x=w375, y=w377) -> (x .or. y?=w378:bool)
              n154 = case shown="False" w378 {
                tunnel: [u8 6 ("Det 3") _] -> w379
                frame False {
                }
                frame True {
                  (unwired) u8 6 ("Det 3")
                }
              }
            }
            frame True {
            }
          }
          n155 = Bundle By Name(cluster=w340, "Latest Correlation"=w333) -> (w360:T16)
          n156 = Bundle By Name(cluster=w352, "Detector Gap Count"=0) -> (w336:T15)
        }
        frame 7 {
          # "q = ADC value / CSA sensitivity"
          # "Ensures the charge is good"
          n157 = Unbundle(w388) -> ("First Correlation"=w402:i32, "Latest Correlation"=w401:i32)
          n158 = Unbundle By Name(w403) -> ("High Charge Limit"=w382:fxp<+,32,-41>, "Low Charge Limit"=w399:fxp<+,32,-41>)
          n159 = Add(x=w402, y=w401) -> (x+y=w391:i32)
          n160 = Increment(x=w386) -> (x+1=w385:T15)
          n161 = Scale By Power Of 2(n=i16 -1, x=w391) -> (x*2^n=w389:i32)
          n162 = To Fixed-Point(number=w389) -> (fixed-point=w390:fxp<+/-,32,32>)  [unwired: 1 in]
          n163 = Multiply(x=w390, y=w400) -> (x*y=w394:fxp<+/-,47,32>)
          n164 = Multiply(x=w394, y=w393) -> (x*y=w384:fxp<+/-,64,-17>)
          n165 = Bundle(cluster=w388, "First Correlation"=w389) -> (w387:T16)  [unwired: 1 in]
          n166 = To Fixed-Point(fixed-point type=w382, number=w384) -> (fixed-point=w383:fxp<+,32,-41>)
          n167 = Less Or Equal?(x=w383, y=w382) -> (x <= y?=w398:bool)
          n168 = Greater Or Equal?(x=w383, y=w399) -> (x >= y?=w397:bool)
          n169 = And(x=w398, y=w397) -> (x .and. y?=w396:bool)
          n170 = case shown="True" w396 {
            tunnel: [u8 8 ("Det 3") _] -> w395
            frame True {
            }
            frame False {
              (unwired) u8 7 ("Det 3")
            }
          }
        }
        frame 8 {
          # "This section ensures that we only look for the particle\nwithin the speed bounds of the current filter"
          n171 = Increment(x=w407) -> (x+1=w406:T15)
          n172 = Unbundle By Name(w413) -> ("Gap Max Speed Count"=w411:i32)
          n173 = Unbundle By Name(w406) -> ("Detector Gap Count"=w412:i32)
          n174 = Greater Or Equal?(x=w412, y=w411) -> (x >= y?=w410:bool)
          n175 = case shown="True" w410 {
            tunnel: [u8 9 u8 8] -> w409
            frame True {
            }
            frame False {
            }
          }
        }
        frame 9 {
          # "Waits for a second detector correlation that's close to the\nfirst correlation, but make sure it's in the right speed range."
          n176 = Unbundle By Name(w419) -> ("First Correlation"=w422:i32)
          n177 = Increment(x=w420) -> (x+1=w417:T15)
          n178 = Unbundle By Name(w430) -> ("Gap Min Speed Count"=w429:i32)
          n179 = Unbundle By Name(w417) -> ("Detector Gap Count"=w421:i32)
          n180 = Add(x=w425, y=w424) -> (x+y=w418:i32)
          n181 = Greater Or Equal?(x=w421, y=w429) -> (x >= y?=w428:bool)
          n182 = case shown="False" w428 {
            tunnel: [_ w445] -> w423
            tunnel: w427 -> [_ w444]
            tunnel: w426 -> [_ w441]
            tunnel: w422 -> [_ w432]
            frame True {
              (unwired) u8 9
            }
            frame False {
              n183 = Unbundle By Name(w441) -> ("Filter 1.Det 2"=w438:i32, "Filter 3.Det 2"=w440:i32, "Filter 4.Det 2"=w439:i32)
              n184 = To Fixed-Point(number=w432) -> (fixed-point=w434:fxp<+/-,32,32>)  [unwired: 1 in]
              n185 = Subtract(x=fxp<+,1,1> 1.0, y=w444) -> (x-y=w442:fxp<+,33,1>)
              n186 = Add(x=w440, y=w439) -> (x+y=w437:i32)
              n187 = Multiply(x=w442, y=w434) -> (x*y=w436:fxp<+/-,64,32>)
              n188 = Subtract(x=w437, y=w438) -> (x-y=w431:i32)
              n189 = To Fixed-Point(number=w431) -> (fixed-point=w433:fxp<+/-,32,32>)  [unwired: 1 in]
              n190 = Greater?(x=w433, y=w436) -> (0:w435:bool)
              n191 = case shown="True" w435 {
                tunnel: [u8 10 u8 9] -> w445
                frame True {
                }
                frame False {
                }
              }
            }
          }
        }
        frame 10 {
          # "Waits for Boxcar 2 to reach the halfway point\nbetween Boxcars 1 and 3+4."
          n192 = Unbundle By Name(w472) -> ("Filter 1.Det 2"=w481:i32, "Filter 3.Det 2"=w484:i32, "Filter 4.Det 2"=w483:i32, "Filter 2.Det 2"=w475:i32)
          n193 = Increment(x=w456) -> (x+1=w451:T15)
          n194 = To Fixed-Point(number=w479) -> (fixed-point=w469:fxp<+/-,32,32>)  [unwired: 1 in]
          n195 = Unbundle By Name(w455) -> ("Gap Min Speed Count"=w453:i32)
          n196 = Unbundle By Name(w456) -> ("Detector Gap Count"=w454:i32)
          n197 = Decrement(x=w487) -> (x-1=w468:i32)
          n198 = Increment(x=w466) -> (x+1=w462:fxp<+,33,1>)
          n199 = Add(x=w484, y=w483) -> (x+y=w482:i32)
          n200 = Unbundle(w465) -> ("First Correlation"=w464:i32)  [unwired: 1 out]
          n201 = To Fixed-Point(number=w464) -> (fixed-point=w463:fxp<+/-,32,32>)  [unwired: 1 in]
          n202 = Add(x=w481, y=w482) -> (x+y=w485:i32)
          n203 = Subtract(x=w482, y=w481) -> (x-y=w461:i32)
          n204 = To Fixed-Point(number=w475) -> (fixed-point=w471:fxp<+/-,32,32>)  [unwired: 1 in]
          n205 = Multiply(x=w463, y=w462) -> (x*y=w459:fxp<+/-,64,33>)
          n206 = To Fixed-Point(number=w478) -> (fixed-point=w470:fxp<+/-,32,32>)  [unwired: 1 in]
          n207 = To Fixed-Point(number=w485) -> (fixed-point=w473:fxp<+/-,32,32>)  [unwired: 1 in]
          n208 = Multiply(x=w473, y=w469) -> (x*y=w480:fxp<+/-,64,64>)
          n209 = To Fixed-Point(number=w461) -> (fixed-point=w460:fxp<+/-,32,32>)  [unwired: 1 in]
          n210 = Scale By Power Of 2(n=i16 1, x=w470) -> (x*2^n=w476:fxp<+/-,32,32>)
          n211 = Greater Or Equal?(x=w454, y=w453) -> (x >= y?=w452:bool)
          n212 = Greater?(x=w460, y=w459) -> (0:w458:bool)
          n213 = Multiply(x=w471, y=w476) -> (x*y=w474:fxp<+/-,64,64>)
          n214 = Or(x=w458, y=w452) -> (x .or. y?=w457:bool)
          n215 = Greater?(x=w480, y=w474) -> (0:w467:bool)
          n216 = case shown="True" w467 {
            tunnel: [w492 u8 11 ("Det 3")] -> w486
            tunnel: w468 -> [w489 _]
            tunnel: w457 -> [w488 _]
            frame False {
              n217 = Less Or Equal To 0?(x=w489) -> (x <= 0?=w490:bool)
              n218 = Or(x=w488, y=w490) -> (x .or. y?=w491:bool)
              n219 = case shown="False" w491 {
                tunnel: [u8 10 ("Det 3") _] -> w492
                frame False {
                }
                frame True {
                  (unwired) u8 10 ("Det 3")
                }
              }
            }
            frame True {
            }
          }
          n220 = Bundle By Name(cluster=w451, "Second Detector Count"=0) -> (w450:T15)
        }
        frame 11 {
          # "This section ensures that we only look for the particle\nwithin the speed bounds of the current filter"
          n221 = Increment(x=w497) -> (x+1=w496:T15)
          n222 = Unbundle By Name(w503) -> ("Detector Max Speed Count"=w501:i32)
          n223 = Unbundle By Name(w496) -> ("Second Detector Count"=w502:i32)
          n224 = Greater Or Equal?(x=w502, y=w501) -> (x >= y?=w500:bool)
          n225 = case shown="True" w500 {
            tunnel: [u8 12 u8 11] -> w499
            frame True {
            }
            frame False {
            }
          }
        }
        frame 12 {
          # "Waits for a reverse correlation that's close to the first correlation, but make sure it's in the right speed range."
          n226 = Unbundle By Name(w520) -> ("Detector Min Speed Count"=w519:i32)
          n227 = Unbundle By Name(w506) -> ("First Correlation"=w512:i32)
          n228 = Increment(x=w510) -> (x+1=w508:T15)
          n229 = Unbundle By Name(w508) -> ("Second Detector Count"=w511:i32)
          n230 = Add(x=w515, y=w514) -> (x+y=w509:i32)
          n231 = Greater Or Equal?(x=w511, y=w519) -> (x >= y?=w518:bool)
          n232 = case shown="False" w518 {
            tunnel: [_ w535] -> w513
            tunnel: w517 -> [_ w534]
            tunnel: w516 -> [_ w531]
            tunnel: w512 -> [_ w522]
            frame True {
              (unwired) u8 12
            }
            frame False {
              n233 = Unbundle By Name(w531) -> ("Filter 1.Det 2"=w528:i32, "Filter 3.Det 2"=w530:i32, "Filter 4.Det 2"=w529:i32)
              n234 = To Fixed-Point(number=w522) -> (fixed-point=w524:fxp<+/-,32,32>)  [unwired: 1 in]
              n235 = Subtract(x=fxp<+,1,1> 1.0, y=w534) -> (x-y=w532:fxp<+,33,1>)
              n236 = Add(x=w530, y=w529) -> (x+y=w527:i32)
              n237 = Multiply(x=w532, y=w524) -> (x*y=w526:fxp<+/-,64,32>)
              n238 = Subtract(x=w528, y=w527) -> (x-y=w521:i32)
              n239 = To Fixed-Point(number=w521) -> (fixed-point=w523:fxp<+/-,32,32>)  [unwired: 1 in]
              n240 = Greater?(x=w523, y=w526) -> (0:w525:bool)
              n241 = case shown="True" w525 {
                tunnel: [u8 13 u8 12] -> w535
                frame True {
                }
                frame False {
                }
              }
            }
          }
        }
        frame 13 {
          # "Waits for Boxcar 2 to reach the halfway point\nbetween Boxcars 1 and 3+4."
          n242 = Unbundle By Name(w545) -> ("Detector Min Speed Count"=w542:i32)
          n243 = Unbundle By Name(w560) -> ("Filter 1.Det 2"=w569:i32, "Filter 3.Det 2"=w572:i32, "Filter 4.Det 2"=w571:i32, "Filter 2.Det 2"=w563:i32)
          n244 = Unbundle By Name(w544) -> ("Second Detector Count"=w543:i32)
          n245 = Increment(x=w544) -> (x+1=w554:T15)
          n246 = To Fixed-Point(number=w567) -> (fixed-point=w557:fxp<+/-,32,32>)  [unwired: 1 in]
          n247 = Decrement(x=w575) -> (x-1=w556:i32)
          n248 = Increment(x=w553) -> (x+1=w550:fxp<+,33,1>)
          n249 = Add(x=w572, y=w571) -> (x+y=w570:i32)
          n250 = Unbundle(w538) -> ("First Correlation"=w552:i32)  [unwired: 1 out]
          n251 = To Fixed-Point(number=w552) -> (fixed-point=w551:fxp<+/-,32,32>)  [unwired: 1 in]
          n252 = Add(x=w569, y=w570) -> (x+y=w573:i32)
          n253 = Subtract(x=w569, y=w570) -> (x-y=w549:i32)
          n254 = To Fixed-Point(number=w563) -> (fixed-point=w559:fxp<+/-,32,32>)  [unwired: 1 in]
          n255 = Multiply(x=w551, y=w550) -> (x*y=w547:fxp<+/-,64,33>)
          n256 = To Fixed-Point(number=w566) -> (fixed-point=w558:fxp<+/-,32,32>)  [unwired: 1 in]
          n257 = To Fixed-Point(number=w573) -> (fixed-point=w561:fxp<+/-,32,32>)  [unwired: 1 in]
          n258 = Greater Or Equal?(x=w543, y=w542) -> (x >= y?=w540:bool)
          n259 = Multiply(x=w561, y=w557) -> (x*y=w568:fxp<+/-,64,64>)
          n260 = To Fixed-Point(number=w549) -> (fixed-point=w548:fxp<+/-,32,32>)  [unwired: 1 in]
          n261 = Scale By Power Of 2(n=i16 1, x=w558) -> (x*2^n=w564:fxp<+/-,32,32>)
          n262 = Greater?(x=w548, y=w547) -> (0:w546:bool)
          n263 = Multiply(x=w559, y=w564) -> (x*y=w562:fxp<+/-,64,64>)
          n264 = Or(x=w546, y=w540) -> (x .or. y?=w541:bool)
          n265 = Less?(x=w568, y=w562) -> (x < y?=w555:bool)
          n266 = case shown="True" w555 {
            tunnel: [w580 u8 14 ("Det 3")] -> w574
            tunnel: w556 -> [w577 _]
            tunnel: w541 -> [w576 _]
            frame False {
              n267 = Less Or Equal To 0?(x=w577) -> (x <= 0?=w578:bool)
              n268 = Or(x=w576, y=w578) -> (x .or. y?=w579:bool)
              n269 = case shown="False" w579 {
                tunnel: [u8 13 ("Det 3") _] -> w580
                frame False {
                }
                frame True {
                  (unwired) u8 13 ("Det 3")
                }
              }
            }
            frame True {
            }
          }
        }
        frame 14 {
          # "Look carefully at the way the Armed variable is treated in here.\nIf One Shot implies Armed (ie, it's okay to let a particle through),\nthe particle is allowed to go through, but Armed is turned off."
          # "v = clockspeed * distance / speed count"
          # "1/2mv^2 = Vq\ntherefore\nm = 2Vq/v^2"
          n270 = Unbundle By Name(w584) -> ("First Detector Count"=w583:i32)
          n271 = Unbundle By Name(w612) -> ("High Velocity Limit"=w599:fxp<+,18,18>, "Low Velocity Limit"=w600:fxp<+,18,18>, "High Mass Limit"=w608:fxp<+,32,-37>, "Low Mass Limit"=w588:fxp<+,32,-37>, "High Voltage"=w603:fxp<+,32,22>)
          n272 = Multiply(x=w603, y=w590) -> (x*y=w609:fxp<+,64,-19>)
          n273 = To Fixed-Point(number=w583) -> (fixed-point=w598:fxp<+/-,32,32>)  [unwired: 1 in]
          n274 = To Fixed-Point(number=w583) -> (fixed-point=w591:fxp<+/-,32,32>)  [unwired: 1 in]
          n275 = Square(x=w591) -> (x^2=w592:fxp<+,63,63>)
          n276 = Multiply(x=w599, y=w598) -> (x*y=w597:fxp<+/-,50,50>)
          n277 = Multiply(x=w598, y=w600) -> (x*y=w596:fxp<+/-,50,50>)
          n278 = Multiply(x=w611, y=w592) -> (x*y=w610:fxp<+,64,19>)
          n279 = To Fixed-Point(fixed-point type=fxp<+,32,-13> 0.0, number=w610) -> (fixed-point=w586:fxp<+,32,-13>)
          n280 = Greater Or Equal?(x=w597, y=w589) -> (x >= y?=w607:bool)
          n281 = Less Or Equal?(x=w596, y=w589) -> (x <= y?=w606:bool)
          n282 = Multiply(x=w609, y=w586) -> (x*y=w593:fxp<+,64,-32>)
          n283 = Scale By Power Of 2(n=i16 1, x=w593) -> (x*2^n=w587:fxp<+,64,-32>)
          n284 = Less Or Equal?(x=w587, y=w608) -> (x <= y?=w605:bool)
          n285 = Greater Or Equal?(x=w587, y=w588) -> (x >= y?=w604:bool)
          n286 = Compound Arithmetic op=AND(w607, w606, w605, w604, w595) -> (w594:bool)
          n287 = case shown="True" w594 {
            tunnel: [u8 15 ("Det 3") _] -> w601
            frame True {
            }
            frame False {
              (unwired) u8 14 ("Det 3")
            }
          }
        }
        frame 15 {
          # "To keep the names in the distance cluster from\ncorrupting the names of the speed counts cluster.\nThis really shouldn't happen, but it does."
          n288 = Unbundle By Name(w623) -> ("First Detector Count"=w629:i32)
          n289 = To Fixed-Point(number=w629) -> (fixed-point=w637:fxp<+/-,32,32>)  [unwired: 1 in]
          n290 = Multiply(x=w637, y=w636) -> (x*y=w635:T20)
          n291 = To Long Integer(number=w635) -> (32bit integer=w634:T21)
          n292 = Scale By Power Of 2(n=i16 -1, x=w627) -> (x*2^n=w628:i32)
          n293 = Subtract(x=w634, y=w633) -> (x-y=w632:T21)
          n294 = Subtract(x=w632, y=w628) -> (x-y=w625:T21)
          n295 = Unbundle By Name(w625) -> ("Distance to PSU"=w622:i32, "Distance to end of PSU"=w621:i32, "Distance to DCS 2"=w620:i32, "Distance to front of LEIL Chamber"=w616:i32, "Distance to DCS 1"=w614:i32)
          n296 = To Long Integer(number=w616) -> (32bit integer=w615:i32)
          n297 = To Long Integer(number=w622) -> (32bit integer=w619:i32)
          n298 = To Long Integer(number=w621) -> (32bit integer=w618:i32)
          n299 = To Long Integer(number=w620) -> (32bit integer=w617:i32)
          n300 = Add(x=w614, y=w630) -> ()  [unwired: 1 out]
          n301 = Bundle(cluster=w623, "First Detector Count"=w619, "Detector Gap Count"=w618, "Second Detector Count"=w617, "Second Detector Final Count"=w615) -> (w624:T15)
        }
        frame 16 {
          n302 = Decrement(x=w664) -> (x-1=w663:T15)
          n303 = Decrement(x=w646) -> (x-1=w639:i32)
          n304 = Unbundle(w663) -> ("First Detector Count"=w660:i32, "Detector Gap Count"=w658:i32, "Second Detector Count"=w655:i32, "Second Detector Final Count"=w653:i32)
          n305 = Add(x=w655, y=w643) -> (x+y=w656:i32)
          n306 = Add(x=w653, y=w643) -> (x+y=w642:i32)
          n307 = Add(x=w639, y=w643) -> (x+y=w641:i32)
          n308 = Less Or Equal To 0?(x=w655) -> (x <= 0?=w654:bool)
          n309 = Greater Or Equal To 0?(x=w642) -> (x >= 0?=w651:bool)
          n310 = Greater Or Equal To 0?(x=w641) -> (x >= 0?=w638:bool)
          n311 = Less Or Equal To 0?(x=w660) -> (x <= 0?=w659:bool)
          n312 = Less Or Equal To 0?(x=w653) -> (x <= 0?=w652:bool)
          n313 = Less Or Equal To 0?(x=w639) -> (x <= 0?=w640:bool)
          n314 = Greater Or Equal To 0?(x=w656) -> (x >= 0?=w648:bool)
          n315 = Greater Or Equal To 0?(x=w658) -> (x >= 0?=w657:bool)
          n316 = And(x=w652, y=w651) -> (x .and. y?=w645:bool)
          n317 = And(x=w640, y=w638) -> (x .and. y?=w644:bool)
          n318 = And(x=w659, y=w657) -> (x .and. y?=w662:bool)
          n319 = And(x=w654, y=w648) -> (x .and. y?=w661:bool)
          n320 = And(x=w647, y=w651) -> (x .and. y?=w649:bool)
          n321 = Compound Arithmetic op=OR(w649, w648, w638) -> (w650:bool)
          n322 = case shown="False" w650 {
            tunnel: [u8 16 ("Det 3") _] -> w665
            frame True {
            }
            frame False {
            }
          }
        }
      }
    }
    n323 = Delete From Array(array=w77) -> (array with subset deleted=w76:cluster{"Det 1":i16, "Det 2":i16}[])  [unwired: 2 in, 1 out]
    n324 = case shown="True" "Calibrate" {
      tunnel: w113 -> [w170 _]
      tunnel: [w170 w171] -> w146
      tunnel: w101 -> [_ w171]
      frame False {
      }
      frame True {
      }
    }
    n325 = Or Array Elements(Boolean array=w123) -> (logical OR=w117:bool)
    n326 = Or Array Elements(Boolean array=w87) -> (logical OR=w93:bool)
    n327 = Or Array Elements(Boolean array=w126) -> (logical OR=w100:bool)
    n328 = Or Array Elements(Boolean array=w125) -> (logical OR=w97:bool)
    n329 = Or Array Elements(Boolean array=w124) -> (logical OR=w95:bool)
    n330 = Not(x=w117) -> (.not. x?=w122:bool)
    n331 = And(x=w122, y=w120) -> (x .and. y?=w121:bool)
    n332 = xnode ("Handshake Write")("Data"=w95, "Input Valid"=TRUE) -> ()  [unwired: 1 in, 2 out]
    n333 = xnode ("Handshake Write")("Data"=w100, "Input Valid"=TRUE) -> ()  [unwired: 1 in, 2 out]
    n334 = local write "Armed"(w121) -> ()
    n335 = xnode ("Handshake Write")("Data"=w97, "Input Valid"=TRUE) -> ()  [unwired: 1 in, 2 out]
    n336 = xnode ("Handshake Write")("Data"=w93, "Input Valid"=TRUE) -> ()  [unwired: 1 in, 2 out]
  }
  n337 = node-c288(w43) -> ()
  n338 = node-c288(w29) -> ()
